vi "CheckLVTimeSync.vi"() -> (0 "error out":errorcluster)   [LabVIEW 2018, in "feGEM DataPacker.lvlib"]
uses:
  feGEM DataPacker.lvlib
  5c77b1e3-c6b4-4847-bd49-cf5dfadfc90b.vi
  5c77b1e3-c6b4-4847-bd49-cf5dfadfc90b.vi/145ec9f3-fa99-4045-8e10-af6dc0ab976a.vi
  <vilib>/Utility/SystemLogging/Write to System Log.vi
panel:
  in  "stop":bool
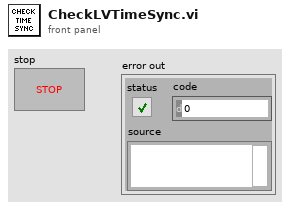
[diagram p1: front panel]
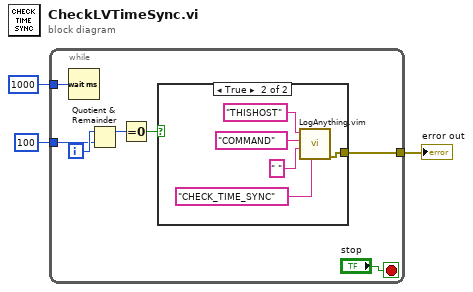
[diagram p0: block diagram]
diagram:
  n1 = while {
    tunnel: u32 1000 ("milliseconds to wait") -> [w9]
    tunnel: [w8] -> w3
    tunnel: u32 100 ("milliseconds to wait") -> [w6]
    i -> [w7]
    stop <- "stop" stop-if-true
    n2 = Wait (ms)(milliseconds to wait=w9) -> ()  [unwired: 1 out]
    n3 = Quotient & Remainder(x=w7, y=w6) -> (x-y*floor(x/y)=w5:u32)  [unwired: 1 out]
    n4 = Equal To 0?(x=w5) -> (x = 0?=w4:bool)
    n5 = case shown="True" w4 {
      tunnel: [_ w15] -> w8
      frame False {
      }
      frame True {
        n6 = call "LogAnything.vim"("Equipment description (32 chars)"="CHECK_TIME_SYNC" ("Category"), "Array"=" ", "Variable Name"="COMMAND" ("Var Name"), "Category"="THISHOST") -> ("error out"=w15:errorcluster)  [unwired: 6 in, 1 out]
      }
    }
  }
  "error out" <- w3
